vi "break number in unit digit_0.vi"() -> ()   [LabVIEW 2015]
panel:
  in  "Tab Control":enum32{"Page 1", "Page 2"}(tab)
  out "Seprate value":dbl[](array[numeric])
  in  "Value":dbl
  out "length":i32
  out "decimal integer string":string
  out "Value 2":dbl
  out "floor(x/y)":dbl
  # "Break a number in unit digit"
  # "Pardeep Kumar"
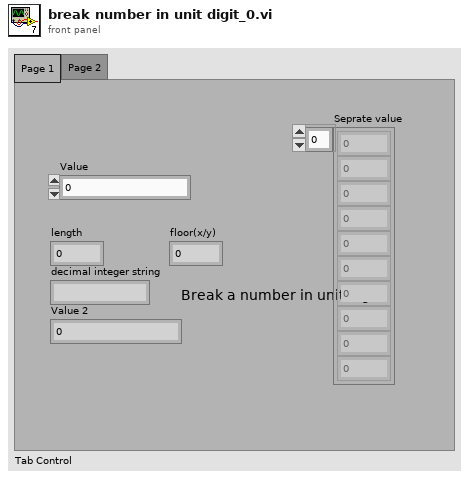
[diagram p1: front panel]
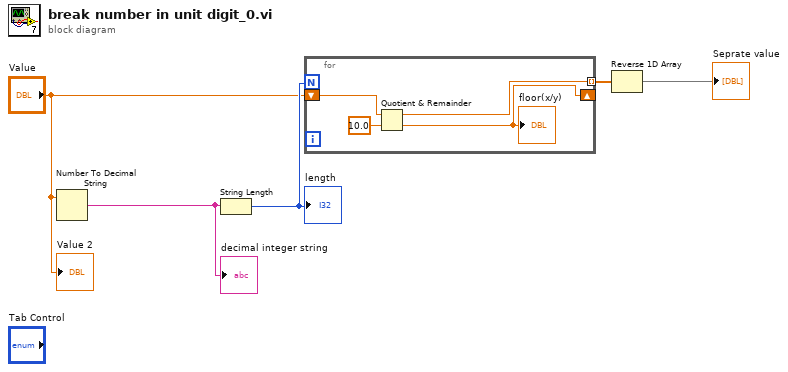
[diagram p0: block diagram]
diagram:
  n1 = Number To Decimal String(number="Value") -> (decimal integer string=w5:string)  [unwired: 1 in]
  "decimal integer string" <- w5
  n2 = String Length(string=w5) -> (length=w4:i32)
  "length" <- w4
  n3 = for {
    N: w4 -> [_]
    tunnel: [w8] -> w2 mode=indexing
    shift-right: [w7] -> _
    shift-left: "Value" -> [w9]
    n4 = Quotient & Remainder(x=w9, y=10.0) -> (x-y*floor(x/y)=w8:dbl, floor(x/y)=w7:dbl)
    "floor(x/y)" <- w7
  }
  n5 = Reverse 1D Array(array=w2) -> (reversed array=→"Seprate value":dbl[])
  "Value 2" <- "Value"
